vi "Read Channel Info.vi"(8 "error in (no error)":errorcluster, 11 "Channel in":refnum<class "Channel.lvclass">) -> (0 "error out":errorcluster, 1 "URL":string, 2 "Name":string, 3 "Channel out":refnum<class "Channel.lvclass">, 4 "DataType":T1, 5 "Read or Write":string)   [LabVIEW 2017, in "Channel.lvlib" / "Channel.lvclass"]
uses:
  Channel.lvclass
  <vilib>/Utility/Data Type/Type Definitions/Data Type.ctl
  Channel.lvclass/Channel.ctl
  <vilib>/Utility/Data Type/NI_Data Type.lvlib
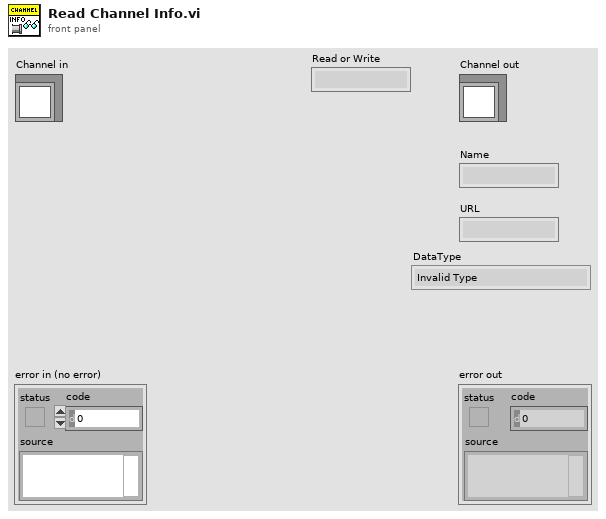
[diagram p1: front panel]
types:
  T1 = typedef "NI_Data Type.lvlib/Data Type.ctl" = enum8{"Invalid Type", "Void", "I8", "I16", "I32", "I64", "U8", "U16", "U32", "U64", "Single Float", "Double Float", "Extended Float", "Single Complex", "Double Complex", "Extended Complex", "Enum U8", "Enum U16", "Enum U32", "Enum U64", "Single Float With Unit", "Double Float With Unit", "Extended Float With Unit", "Single Complex with Unit", "Double Complex with Unit", "Extended Complex with Unit", "Boolean", "String", "Path", "Picture", "Tag", "Array", "Cluster", "Variant", "LV Variant", "Waveform", "Timestamp", "Digital Waveform", "Digital Data", "ExpressData", "Refnum", "External Data", "VI", "Poly VI", "LabVIEW Class Instance", "Fixed Point"}
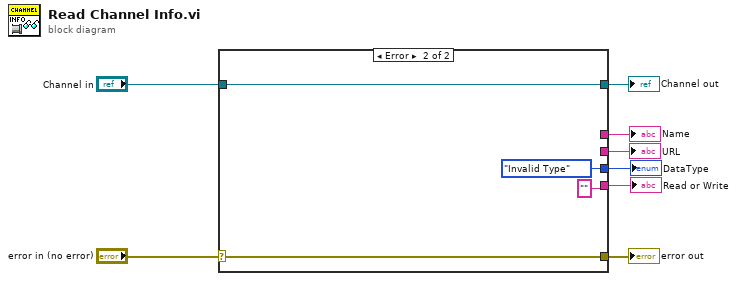
[diagram p0: block diagram]
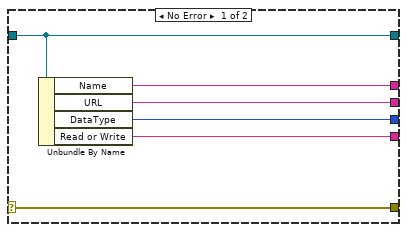
[diagram p2: hidden frame]
diagram:
  n1 = case shown="Error" "error in (no error)" {
    selector: "error in (no error)" -> [w14 w17]
    tunnel: [w14 w17] -> w7
    tunnel: [w13 w18] -> w5
    tunnel: "Channel in" -> [w13 w18]
    tunnel: [w12 _] -> w4
    tunnel: [w11 _] -> w3
    tunnel: [w10 "" ("Read or Write")] -> w2
    tunnel: [w9 Data_Type."Invalid Type" ("DataType")] -> w1
    frame No Error {
      n2 = Unbundle By Name(w13) -> ("Name"=w12:string, "URL"=w11:string, "DataType"=w9:T1, "Read or Write"=w10:string)
    }
    frame Error {
    }
  }
  "error out" <- w7
  "Channel out" <- w5
  "Name" <- w4
  "URL" <- w3
  "Read or Write" <- w2
  "DataType" <- w1
